vi "Read Selection.vi"(8 "error in (no error)":errorcluster, 11 "Dialog_2Buttons.lvclass in":refnum<class "Dialog_TwoButtons.lvclass">) -> (0 "error out":errorcluster, 2 "Selection (-1: none)":i8=-1, 3 "Dialog_2Buttons.lvclass out":refnum<class "Dialog_TwoButtons.lvclass">)   [LabVIEW 2012, in "Dialog_TwoButtons.lvlib" / "Dialog_TwoButtons.lvclass"]
doc: "Accessor VI for Dialog_2Button class"
uses:
  Dialog_TwoButtons.lvclass
  Dialog_TwoButtons.lvclass/Dialog_TwoButtons.ctl
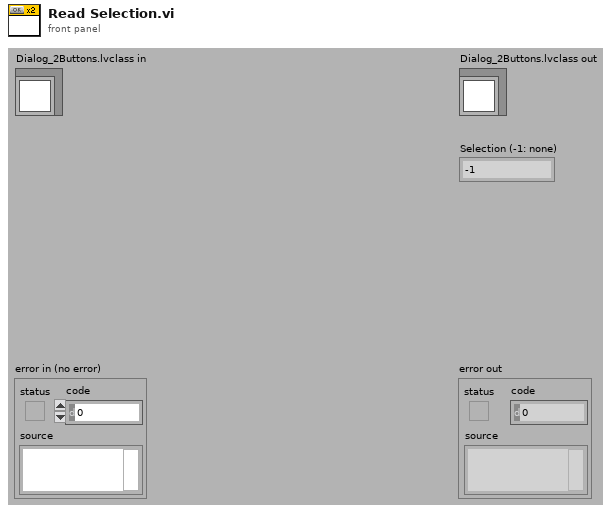
[diagram p1: front panel]
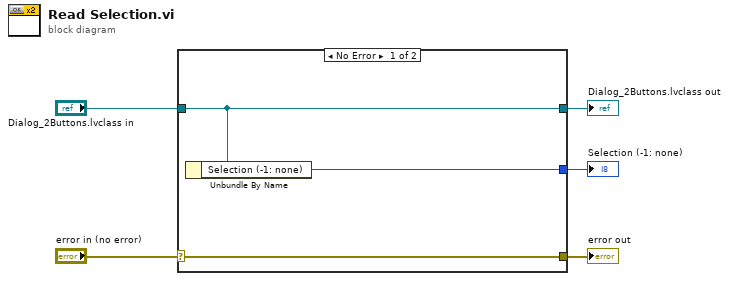
[diagram p0: block diagram]
diagram:
  n1 = case shown="No Error" "error in (no error)" {
    selector: "error in (no error)" -> [w8 w9]
    tunnel: [w8 w9] -> w4
    tunnel: [w7 w10] -> w2
    tunnel: "Dialog_2Buttons.lvclass in" -> [w7 w10]
    tunnel: [w6 _] -> w1
    frame No Error {
      n2 = Unbundle By Name(w7) -> ("Selection (-1: none)"=w6:i8)
    }
    frame Error {
    }
  }
  "error out" <- w4
  "Dialog_2Buttons.lvclass out" <- w2
  "Selection (-1: none)" <- w1
